vi "RTS Macro Look For Resistance Heater.vi"(0 "Refrigeration Full Data Output":T2, 5 "Refrigeration Core Stats Input":T1 {"Average Compressor Cycle Time (Min)" format="%0.2f"; "Average Compressor Power (W)" format="%0.2f"; "Power Start Time (sec)" format="%<%H:%M:%S>t"; "Power End time (sec)" format="%<%H:%M:%S>t"; "Average Defrost Power (W)" format="%0.2f"}, 11 "Error In":errorcluster, 12 "Average Compressor Power (Lower)":dbl=10.0 format="%#_13g") -> (3 "Power Compressor Run 2":cluster{dbl[], dbl[]}(graph), 4 "Time Array":dbl[](array[numeric]), 6 "Refrigeration Core Stats Output":T1 {"Average Compressor Cycle Time (Min)" format="%0.2f"; "Average Compressor Power (W)" format="%0.2f"; "Power Start Time (sec)" format="%<%H:%M:%S>t"; "Power End time (sec)" format="%<%H:%M:%S>t"; "Average Defrost Power (W)" format="%0.2f"}, 15 "Error Out":errorcluster)   [LabVIEW 2016]
uses:
  Type Definitions/RTS Macro Full Data.ctl
  Type Definitions/RTS Macro Refrigeration Core Stats.ctl
  <vilib>/Analysis/baseanly.llb/Mean (DBL).vi
  <vilib>/Analysis/NI_AALBase.lvlib
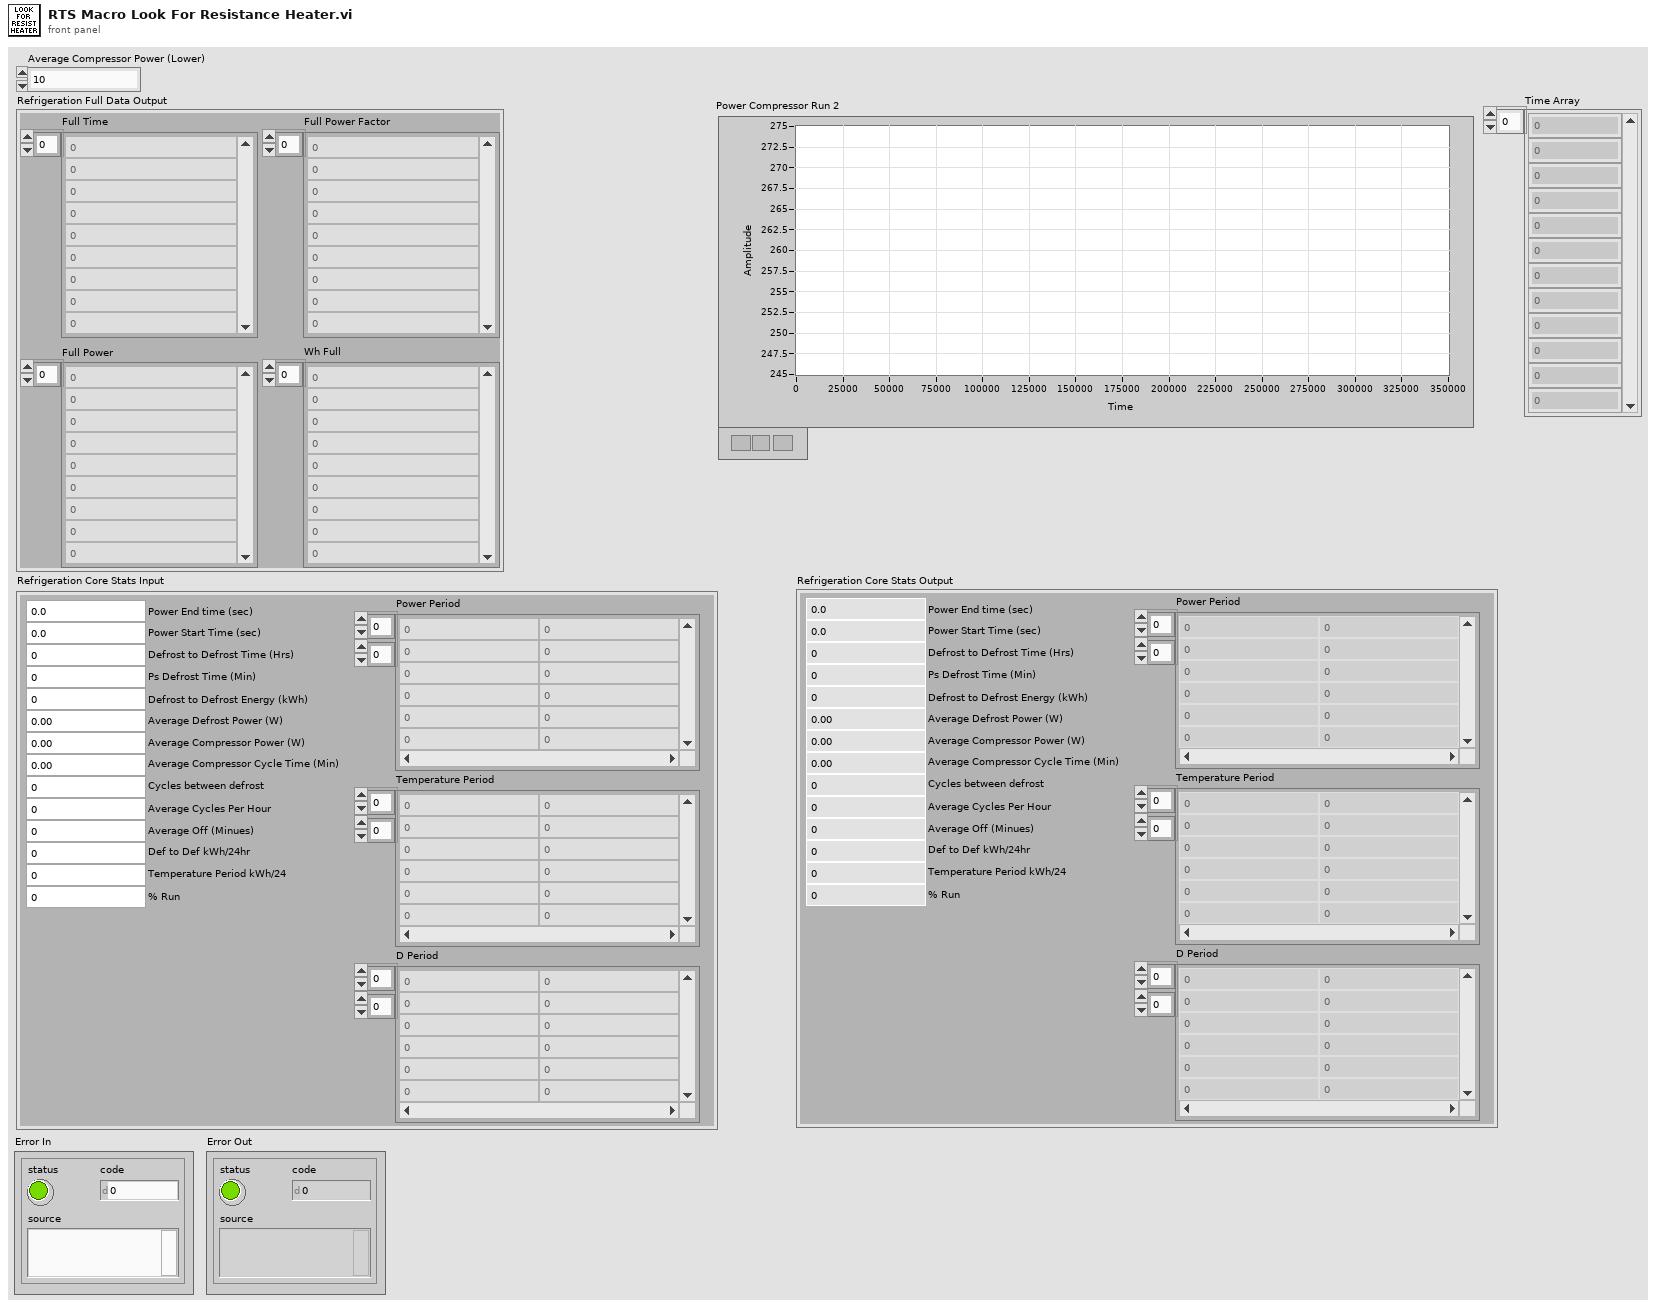
[diagram p1: front panel]
types:
  T1 = typedef "RTS Macro Refrigeration Core Stats.ctl" = cluster{"Average Defrost Power (W)":dbl, "Power End time (sec)":dbl, "Power Start Time (sec)":dbl, "Defrost to Defrost Time (Hrs)":dbl, "Ps Defrost Time (Min)":dbl, "Defrost to Defrost Energy (kWh)":dbl, "Average Compressor Power (W)":dbl, "Average Compressor Cycle Time (Min)":dbl, "Power Period":dbl[][], "Cycles between defrost":i32, "Average Cycles Per Hour":dbl, "Average Off (Minues)":dbl, "Def to Def kWh/24hr":dbl, "Temperature Period kWh/24":dbl, "% Run":dbl, "Temperature Period":dbl[][], "D Period":dbl[][]}
  T2 = typedef "RTS Macro Full Data.ctl" = cluster{"Full Time":dbl[], "Full Power Factor":dbl[], "Full Power":dbl[], "Wh Full":dbl[]}
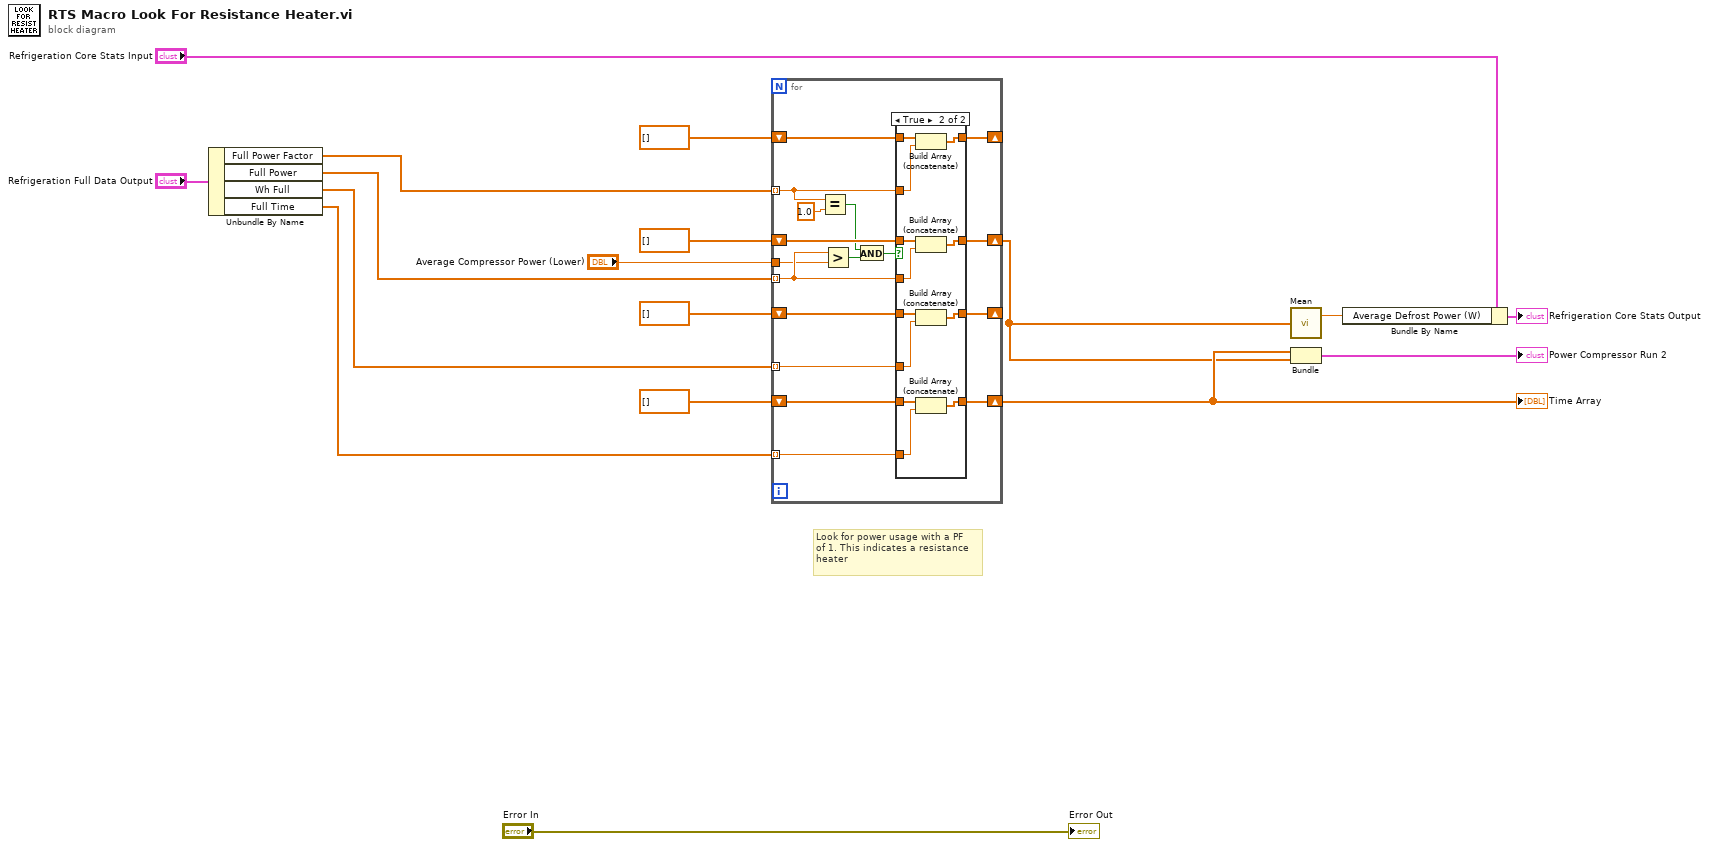
[diagram p0: block diagram]
diagram:
  # "Look for power usage with a PF\nof 1. This indicates a resistance \nheater"
  n1 = Unbundle By Name("Refrigeration Full Data Output") -> ("Full Power Factor"=w4:dbl[], "Full Power"=w5:dbl[], "Wh Full"=w6:dbl[], "Full Time"=w7:dbl[])
  n2 = for {
    tunnel: w4 -> [w24] mode=indexing
    shift-right: [w33] -> _
    shift-left: dbl[] [] -> [w34]
    shift-right: [w31] -> w9
    shift-left: dbl[] [] -> [w32]
    tunnel: w5 -> [w22] mode=indexing
    shift-right: [w29] -> _
    shift-left: dbl[] [] -> [w30]
    tunnel: w6 -> [w28] mode=indexing
    tunnel: w7 -> [w25] mode=indexing
    shift-right: [w26] -> w17
    shift-left: dbl[] [] -> [w27]
    tunnel: "Average Compressor Power (Lower)" -> [w18]
    n3 = Equal?(x=w24, y=1.0) -> (x = y?=w20:bool)
    n4 = Greater?(x=w22, y=w18) -> (0:w21:bool)
    n5 = And(x=w20, y=w21) -> (x .and. y?=w19:bool)
    n6 = case shown="True" w19 {
      tunnel: w34 -> [w38 w50]
      tunnel: [w38 w49] -> w33
      tunnel: w24 -> [_ w48]
      tunnel: w32 -> [w37 w47]
      tunnel: [w37 w46] -> w31
      tunnel: w22 -> [_ w45]
      tunnel: w30 -> [w36 w44]
      tunnel: [w36 w43] -> w29
      tunnel: w28 -> [_ w42]
      tunnel: w27 -> [w35 w41]
      tunnel: [w35 w40] -> w26
      tunnel: w25 -> [_ w39]
      frame False {
      }
      frame True {
        n7 = Build Array (concatenate)(w50, w48) -> (w49:dbl[])
        n8 = Build Array (concatenate)(w47, w45) -> (w46:dbl[])
        n9 = Build Array (concatenate)(w44, w42) -> (w43:dbl[])
        n10 = Build Array (concatenate)(w41, w39) -> (w40:dbl[])
      }
    }
  }
  "Time Array" <- w17
  n11 = call-poly <vilib>:"Mean.vi"("X"=w9) -> ("mean"=w2:dbl)  [unwired: 1 out]
  n12 = Bundle(w17, w9) -> (→"Power Compressor Run 2":cluster{dbl[], dbl[]})  [unwired: 1 in]
  n13 = Bundle By Name(cluster="Refrigeration Core Stats Input", "Average Defrost Power (W)"=w2) -> (→"Refrigeration Core Stats Output":T1)
  "Error Out" <- "Error In"
